vi "Update used channels.vi"(8 "error in (no error)":errorcluster, 10 "Used DAQ Channels in":tag[](array[tag]), 11 "UI in":refnum<class "UI.lvclass">) -> (0 "error out":errorcluster, 3 "UI out":refnum<class "UI.lvclass">)   [LabVIEW 2015, in "UI.lvlib" / "UI.lvclass"]
uses:
  UI.lvclass
  UI.lvclass/UI.ctl
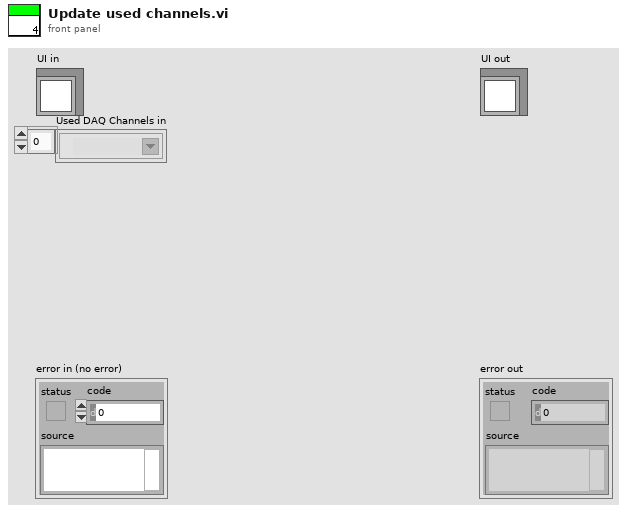
[diagram p1: front panel]
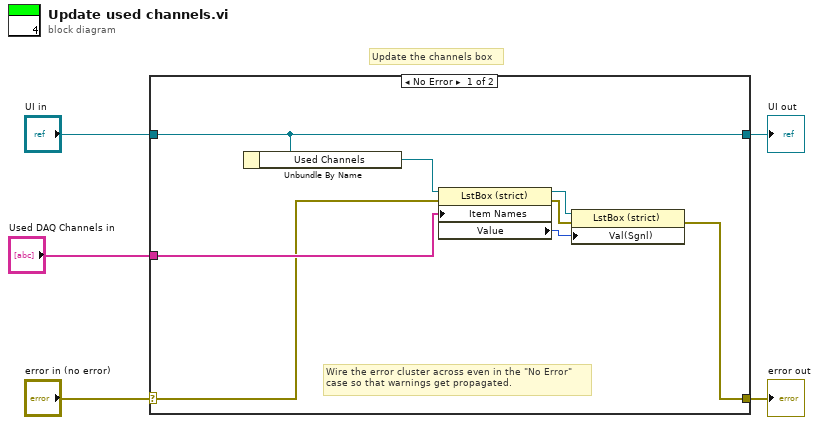
[diagram p0: block diagram]
diagram:
  # "Update the channels box"
  n1 = case shown="No Error" "error in (no error)" {
    selector: "error in (no error)" -> [w10 w15]
    tunnel: [w6 w15] -> w4
    tunnel: [w13 w14] -> w2
    tunnel: "UI in" -> [w13 w14]
    tunnel: "Used DAQ Channels in" -> [w11 _]
    frame No Error {
      # "Wire the error cluster across even in the \"No Error\"\ncase so that warnings get propagated."
      n2 = Unbundle By Name(w13) -> ("Used Channels"=w12:refnum<vi>)
      n3 = property class="LstBox (strict)"(reference=w12, error in=w10, "Item Names"=w11) -> (reference out=w8:refnum<vi>, error out=w7:errorcluster, "Value"=w9:i32)
      n4 = property class="LstBox (strict)"(reference=w8, error in=w7, "Val(Sgnl)"=w9) -> (error out=w6:errorcluster)  [unwired: 1 out]
    }
    frame Error {
    }
  }
  "error out" <- w4
  "UI out" <- w2
